vi "I_O visa.vi"(1 "byte count":i32=4096, 7 "data to write":string="READ:SYS:CAT", 8 "error in":errorcluster, 11 "VISA resource name":refnum<visa-resource-name>) -> (0 "error out":errorcluster, 2 "read data":string, 3 "VISA resource name out":refnum<visa-resource-name>)   [LabVIEW 2013]
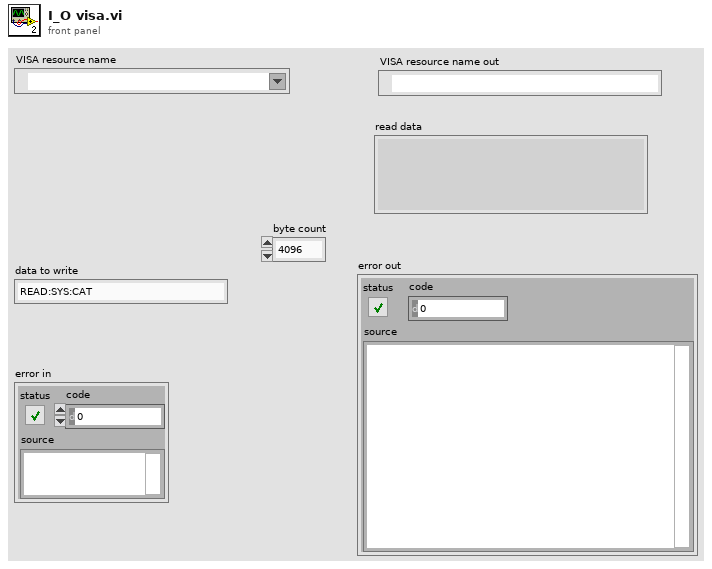
[diagram p1: front panel]
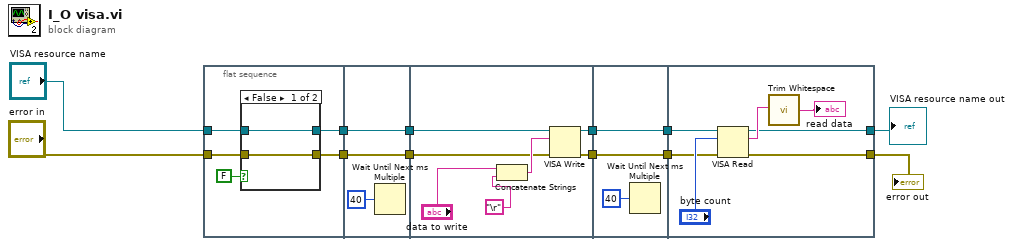
[diagram p0: block diagram]
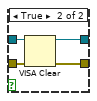
[diagram p2: hidden frame]
diagram:
  n1 = flat-sequence {
    tunnel: "VISA resource name" -> [w17]
    tunnel: "error in" -> [w16]
    tunnel: [w14] -> w2
    tunnel: [w15] -> w1
    tunnel: [w26] -> w4
    tunnel: [w25] -> w3
    tunnel: w2 -> [w26]
    tunnel: w1 -> [w25]
    tunnel: [w33] -> w12
    tunnel: [w32] -> w9
    tunnel: w4 -> [w28]
    tunnel: w3 -> [w27]
    tunnel: [w35] -> w11
    tunnel: w12 -> [w35]
    tunnel: [w34] -> w10
    tunnel: w9 -> [w34]
    tunnel: w11 -> [w42]
    tunnel: w10 -> [w41]
    tunnel: [w38] -> w8
    tunnel: [w37] -> w7
    frame #0 {
      n2 = case shown="False" FALSE {
        tunnel: w17 -> [w19 w23]
        tunnel: w16 -> [w18 w22]
        tunnel: [w19 w21] -> w15
        tunnel: [w18 w20] -> w14
        frame False {
        }
        frame True {
          n3 = VISA Clear(VISA resource name=w23, error in (no error)=w22) -> (VISA resource name out=w21:refnum<visa-resource-name>, error out=w20:errorcluster)
        }
      }
    }
    frame #1 {
      n4 = Wait Until Next ms Multiple(millisecond multiple=u32 40) -> ()  [unwired: 1 out]
    }
    frame #2 {
      n5 = Concatenate Strings("data to write", "\r") -> (w29:string)
      n6 = VISA Write(VISA resource name=w27, write buffer=w29, error in (no error)=w28) -> (VISA resource name out=w32:refnum<visa-resource-name>, error out=w33:errorcluster)  [unwired: 1 out]
    }
    frame #3 {
      n7 = Wait Until Next ms Multiple(millisecond multiple=u32 40) -> ()  [unwired: 1 out]
    }
    frame #4 {
      n8 = VISA Read(VISA resource name=w41, byte count="byte count", error in (no error)=w42) -> (VISA resource name out=w38:refnum<visa-resource-name>, read buffer=w40:string, error out=w37:errorcluster)  [unwired: 1 out]
      n9 = call <vilib>:"Trim Whitespace.vi"("string"=w40) -> ("trimmed string"=→"read data":string)  [unwired: 1 in]
    }
  }
  "VISA resource name out" <- w8
  "error out" <- w7
